vi "LV2OO Style Global_Reentrant.vi"(2 "error in (no error)":errorcluster, 3 "Action in":refnum<class "Action.lvclass">) -> (0 "error out":errorcluster, 1 "Action out":refnum<class "Action.lvclass">)   [LabVIEW 2014]
uses:
  Action/Action.lvclass
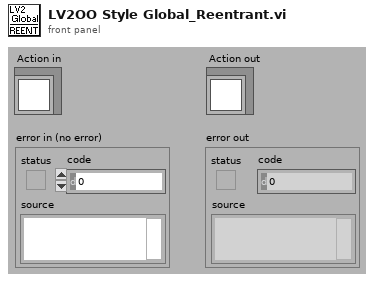
[diagram p1: front panel]
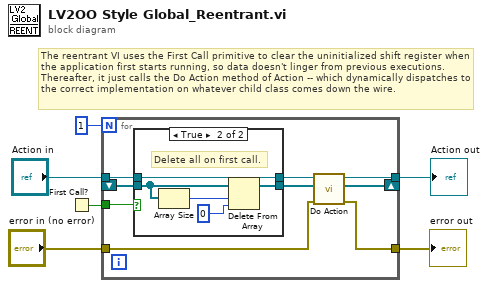
[diagram p0: block diagram]
diagram:
  # "The reentrant VI uses the First Call primitive to clear the uninitialized shift register when the application first starts running, so data doesn't linger from previous executions. Thereafter, it just calls the Do Action method of Action -- which dynamically dispatches to the correct implementation on whatever child class comes down the wire."
  n1 = First Call?() -> (First Call?: T/F=w1:bool)
  n2 = for {
    N: 1 -> [_]
    shift-right: [w14] -> _
    shift-left: _ -> [w9]
    tunnel: "Action in" -> [w10]
    tunnel: [w15] -> w2
    tunnel: "error in (no error)" -> [w13]
    tunnel: [w12] -> w3
    tunnel: w1 -> [w7]
    n3 = case shown="True" w7 {
      tunnel: [w17 w22] -> w11
      tunnel: w10 -> [w17 w22]
      tunnel: w9 -> [w16 w20]
      tunnel: [w16 w21] -> w8
      frame False {
      }
      frame True {
        # "Delete all on first call."
        n4 = Array Size(array=w20) -> (size(s)=w19:i32)
        n5 = Delete From Array(array=w20, length=w19, index=0) -> (array with subset deleted=w21:refnum<class>[])  [unwired: 1 out]
      }
    }
    n6 = call-dynamic "Do Action.vi"("error in (no error)"=w13, "Array in"=w8, "Action in"=w11) -> ("error out"=w12:errorcluster, "Array out"=w14:refnum<class>[], "Action out"=w15:refnum<class "Action.lvclass">)  [unwired: 2 in]
  }
  "error out" <- w3
  "Action out" <- w2
